vi "SimplePassReceiverRole.vi"(6 "first call":bool, 7 "Game in":refnum<class "Game.lvclass">, 8 "error in (no error)":errorcluster, 10 "Tactic index in":i32, 11 "SimplePassReceiverRole in":refnum<class "SimplePassReceiverRole.lvclass">) -> (0 "error out":errorcluster, 1 "tactic index":i32, 2 "Robot out":refnum<class "Robot.lvclass">, 3 "SimplePassReceiverRole out":refnum<class "SimplePassReceiverRole.lvclass">)   [LabVIEW 2018, in "SimplePassReceiverRole.lvclass"]
uses:
  SimplePassReceiverRole.lvclass
  Game_class/Game.lvclass
  Robot_class/Robot.lvclass
  Role_class/Role.lvclass/Role.ctl
  Tacticbook_class/Tacticbook.lvclass/Tacticbook.ctl
  HaltTactic_class/HaltTactic.lvclass/HaltTactic.ctl
  ShootTactic_class/States.ctl
  ShootTactic_class/ShootTactic.lvclass/ShootTactic.ctl
  Tacticbook_class/Read WaitRollTatic.vi
  Tacticbook_class/Write WaitRollTatic.vi
  Tacticbook_class/Read HaltTactic.vi
  HaltTactic_class/Read States.vi
  Tacticbook_class/Write HaltTactic.vi
  Tacticbook_class/Read ShootTactic.vi
  ShootTactic_class/Read States.vi
  Tacticbook_class/Write ShootTactic.vi
  Role_class/Read Tacticbook.vi
  Role_class/Write Tacticbook.vi
  Role_class/Write tactic_index.vi
  Role_class/Read RobotRef.vi
  Tacticbook_class/Tacticbook.lvclass
  WaitRollTatic_class/WaitRollTatic.lvclass
  HaltTactic_class/HaltTactic.lvclass
  ShootTactic_class/ShootTactic.lvclass
panel:
  out "Game out":refnum<class "Game.lvclass">
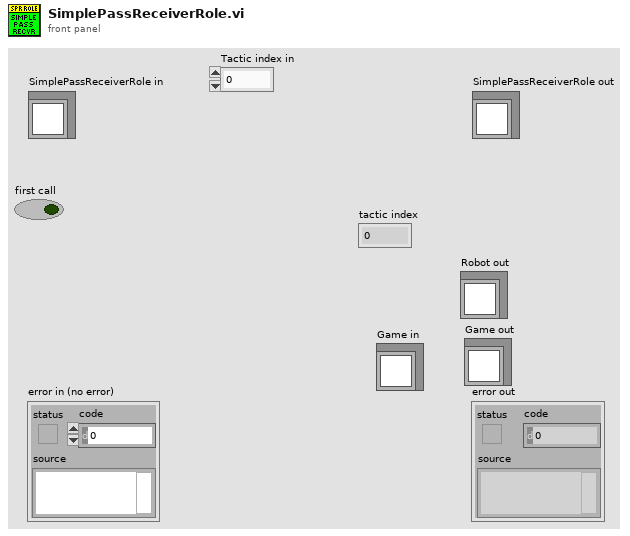
[diagram p1: front panel]
types:
  T1 = typedef "ShootTactic.lvclass/States.ctl" = enum16{"BallInGoalieArea", "Exit", "KickToGoal", "StealBall"}
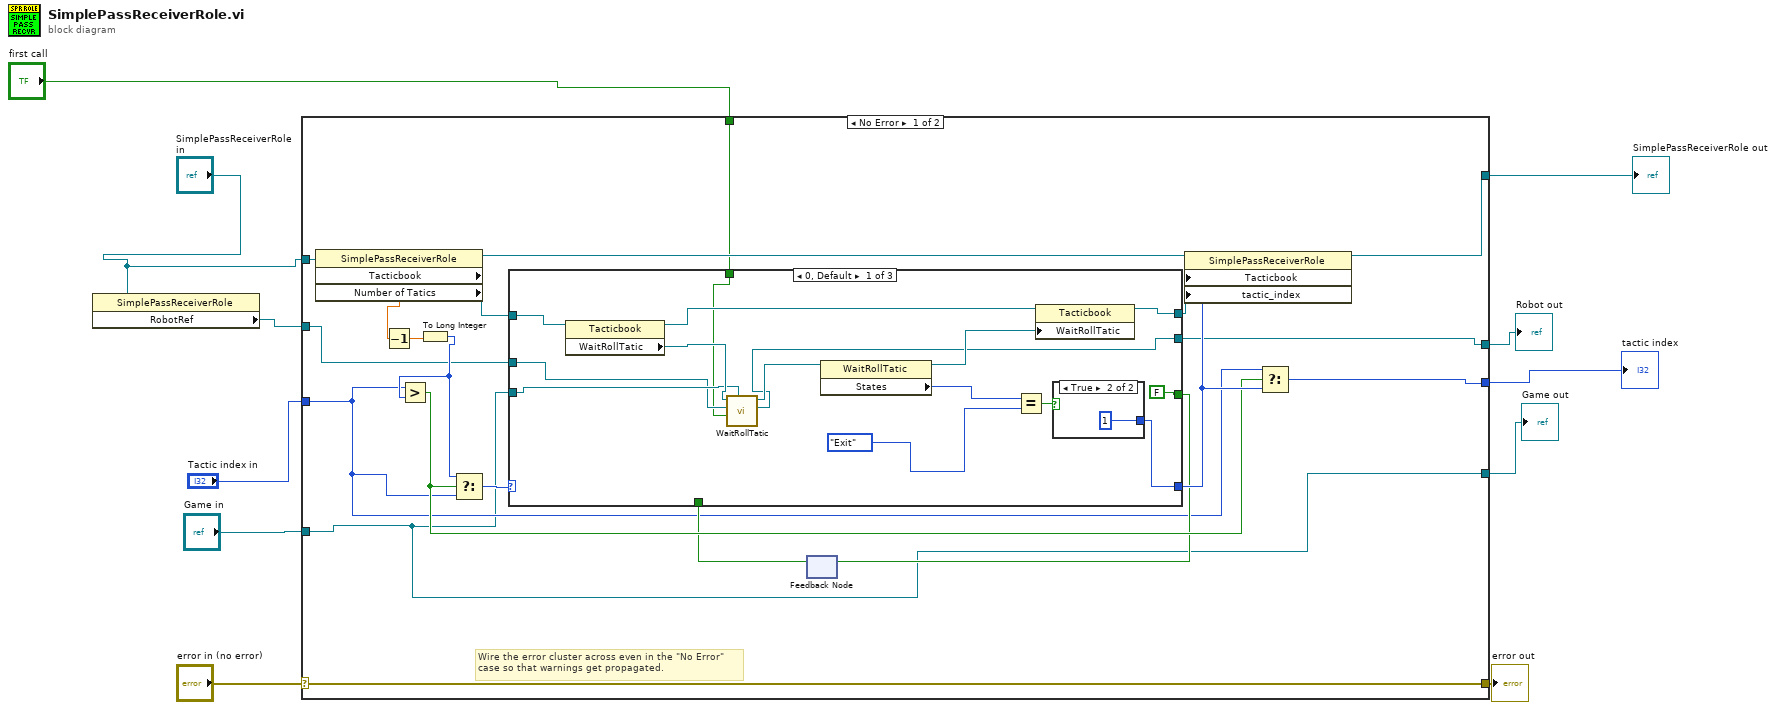
[diagram p0: block diagram]
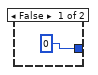
[diagram p2: hidden frame]
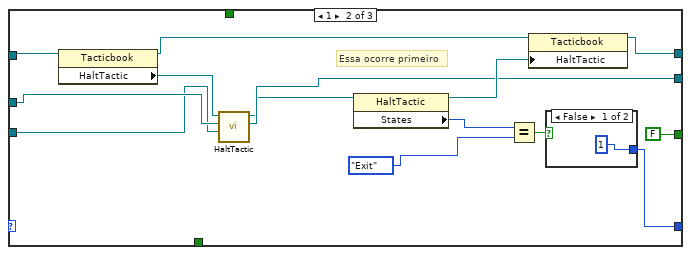
[diagram p3: hidden frame]
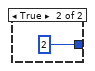
[diagram p4: hidden frame]
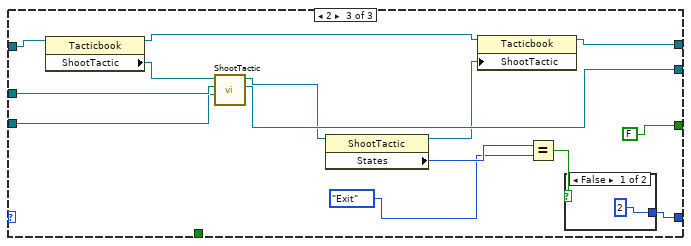
[diagram p5: hidden frame]
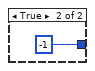
[diagram p6: hidden frame]
diagram:
  n1 = property class="SimplePassReceiverRole"(reference="SimplePassReceiverRole in") -> ("RobotRef"=w9:refnum<class "Robot.lvclass">)  [unwired: 1 in, 2 out]
  n2 = case shown="No Error" "error in (no error)" {
    selector: "error in (no error)" -> [w31 w85]
    tunnel: [w31 w85] -> w10
    tunnel: "SimplePassReceiverRole in" -> [w20 w84]
    tunnel: w9 -> [w19 w83]
    tunnel: "first call" -> [w18 _]
    tunnel: [w17 w84] -> w7
    tunnel: "Tactic index in" -> [w15 w82]
    tunnel: "Game in" -> [w12 w81]
    tunnel: [w14 w83] -> w4
    tunnel: [w13 w82] -> w3
    tunnel: [w12 w81] -> w2
    frame No Error {
      # "Wire the error cluster across even in the \"No Error\"\ncase so that warnings get propagated."
      n3 = property class="SimplePassReceiverRole"(reference=w20) -> (reference out=w30:refnum<class "SimplePassReceiverRole.lvclass">, "Tacticbook"=w29:refnum<class "Tacticbook.lvclass">, "Number of Tatics"=w16:dbl)  [unwired: 1 in, 1 out]
      n4 = Decrement(x=w16) -> (x-1=w22:dbl)
      n5 = To Long Integer(number=w22) -> (32bit integer=w21:i32)
      n6 = Greater?(x=w15, y=w21) -> (0:w25:bool)
      n7 = Select(t=w21, s=w25, f=w15) -> (s? t:f=w26:i32)
      n8 = feedback #1() -> (w23:bool)  [unwired: 1 in]
      n9 = case shown="0, Default" w26 {
        tunnel: [w40 w57 w66] -> w27
        tunnel: w29 -> [w44 w55 w78]
        tunnel: w19 -> [w36 w53 w76]
        tunnel: [w34 w51 w74] -> w14
        tunnel: [w42 w60 w69] -> w28
        tunnel: w12 -> [w37 w52 w75]
        tunnel: w18 -> [w33 _ _]
        tunnel: [FALSE FALSE FALSE] -> w24
        tunnel: w23 -> [_ _ _]
        frame 0, Default {
          n10 = property class="Tacticbook"(reference=w44) -> (reference out=w43:refnum<class "Tacticbook.lvclass">, "WaitRollTatic"=w38:refnum<class "WaitRollTatic.lvclass">)  [unwired: 1 in, 1 out]
          n11 = call "WaitRollTatic.vi"("Game in"=w37, "first call"=w33, "Robot"=w36, "WaitRollTatic in"=w38) -> ("Robot out"=w34:refnum<class "Robot.lvclass">, "WaitRollTatic out"=w35:refnum<class "WaitRollTatic.lvclass">)  [unwired: 5 in, 1 out]
          n12 = property class="WaitRollTatic"(reference=w35) -> (reference out=w41:refnum<class "WaitRollTatic.lvclass">, "States"=w45:enum16{"WaitRoll", "Halt", "Exit"})  [unwired: 1 in, 1 out]
          n13 = Equal?(x=w45, y=enum16{"WaitRoll", "Halt", "Exit"}."Exit" ("States")) -> (x = y?=w46:bool)
          n14 = property class="Tacticbook"(reference=w43, "WaitRollTatic"=w41) -> (reference out=w42:refnum<class "Tacticbook.lvclass">)  [unwired: 1 in, 1 out]
          n15 = case shown="True" w46 {
            tunnel: [0 1] -> w40
            frame False {
            }
            frame True {
            }
          }
        }
        frame 1 {
          # "Essa ocorre primeiro"
          n16 = property class="Tacticbook"(reference=w55) -> (reference out=w62:refnum<class "Tacticbook.lvclass">, "HaltTactic"=w54:refnum<class "HaltTactic.lvclass">)  [unwired: 1 in, 1 out]
          n17 = call-dynamic "HaltTactic.vi"("Game in"=w52, "Robot"=w53, "HaltTactic in"=w54) -> ("Robot out"=w51:refnum<class "Robot.lvclass">, "HaltTactic out"=w50:refnum<class "HaltTactic.lvclass">)  [unwired: 6 in, 1 out]
          n18 = property class="HaltTactic"(reference=w50) -> (reference out=w61:refnum<class "HaltTactic.lvclass">, "States"=w58:enum16{"Halt", "Exit"})  [unwired: 1 in, 1 out]
          n19 = Equal?(x=w58, y=enum16{"Halt", "Exit"}."Exit" ("States")) -> (x = y?=w59:bool)
          n20 = property class="Tacticbook"(reference=w62, "HaltTactic"=w61) -> (reference out=w60:refnum<class "Tacticbook.lvclass">)  [unwired: 1 in, 1 out]
          n21 = case shown="False" w59 {
            tunnel: [1 2] -> w57
            frame False {
            }
            frame True {
            }
          }
        }
        frame 2 {
          n22 = property class="Tacticbook"(reference=w78) -> (reference out=w70:refnum<class "Tacticbook.lvclass">, "ShootTactic"=w77:refnum<class "ShootTactic.lvclass">)  [unwired: 1 in, 1 out]
          n23 = call "ShootTactic.vi"("Game in"=w75, "Robot"=w76, "ShootTactic in"=w77) -> ("Robot out"=w74:refnum<class "Robot.lvclass">, "ShootTactic out"=w71:refnum<class "ShootTactic.lvclass">)  [unwired: 6 in, 1 out]
          n24 = property class="ShootTactic"(reference=w71) -> (reference out=w68:refnum<class "ShootTactic.lvclass">, "States"=w72:T1)  [unwired: 1 in, 1 out]
          n25 = property class="Tacticbook"(reference=w70, "ShootTactic"=w68) -> (reference out=w69:refnum<class "Tacticbook.lvclass">)  [unwired: 1 in, 1 out]
          n26 = Equal?(x=w72, y=States."Exit" ("States")) -> (x = y?=w73:bool)
          n27 = case shown="False" w73 {
            tunnel: [2 -1] -> w66
            frame False {
            }
            frame True {
            }
          }
        }
      }
      n28 = feedback-in #1(w24) -> ()
      n29 = property class="SimplePassReceiverRole"(reference=w30, "Tacticbook"=w28, "tactic_index"=w27) -> (reference out=w17:refnum<class "SimplePassReceiverRole.lvclass">)  [unwired: 1 in, 1 out]
      n30 = Select(t=w15, s=w25, f=w27) -> (s? t:f=w13:i32)
    }
    frame Error {
    }
  }
  "error out" <- w10
  "SimplePassReceiverRole out" <- w7
  "Robot out" <- w4
  "Game out" <- w2
  "tactic index" <- w3
